vi "当前路径.vi"() -> (0 "路径":path)   [LabVIEW 2012]
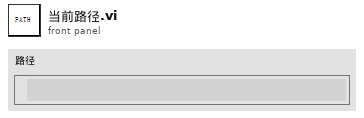
[diagram p1: front panel]
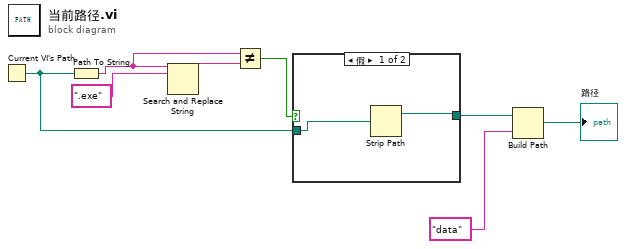
[diagram p0: block diagram]
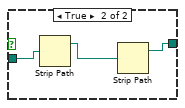
[diagram p2: hidden frame]
diagram:
  n1 = Current VI's Path() -> (path=w4:path)
  n2 = Path To String(path=w4) -> (string=w8:string)
  n3 = Search and Replace String(input string=w8, search string=".exe") -> (result string=w7:string)  [unwired: 6 in, 3 out]
  n4 = Not Equal?(x=w8, y=w7) -> (x != y?=w5:bool)
  n5 = case shown="假" w5 {
    tunnel: w4 -> [w10 w13]
    tunnel: [w9 w11] -> w3
    frame False {
      n6 = Strip Path(path=w10) -> (stripped path=w9:path)  [unwired: 1 out]
    }
    frame True {
      n7 = Strip Path(path=w13) -> (stripped path=w12:path)  [unwired: 1 out]
      n8 = Strip Path(path=w12) -> (stripped path=w11:path)  [unwired: 1 out]
    }
  }
  n9 = Build Path(base path=w3, name or relative path="data") -> (appended path=→"路径":path)
